vi "Picture_shrNonLin_Save_to_matlab.vi"   [LabVIEW 2011]
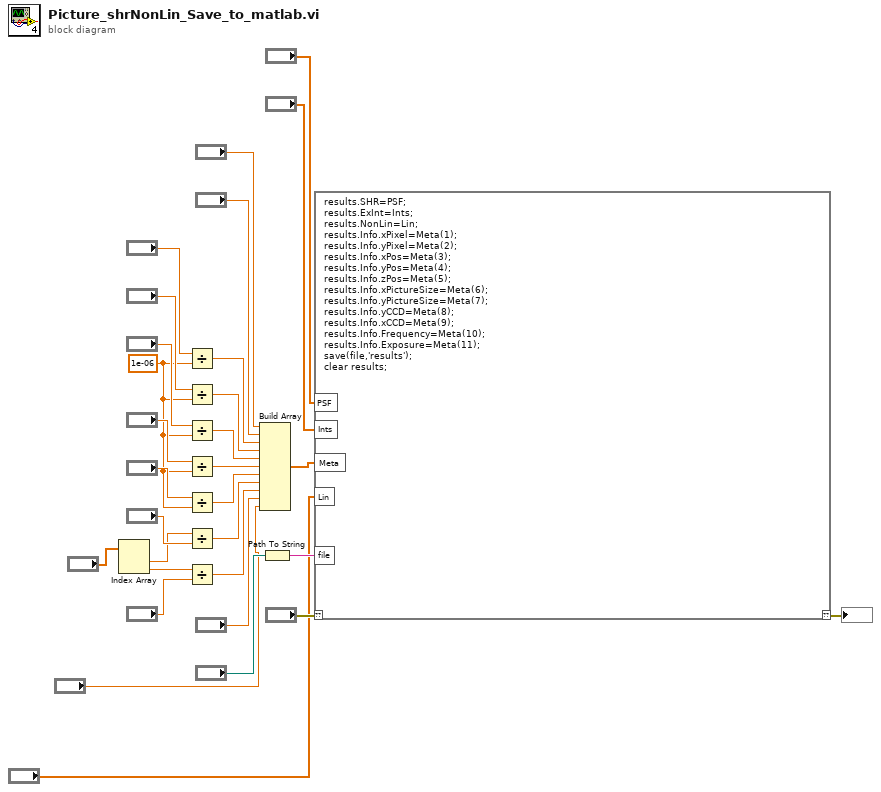
[diagram p0: block diagram]
diagram:
  w9 = 1e-06 ("y")
  n1 = Index Array(array="?") -> (element #1=w4:dbl, element #2=w5:dbl)  [unwired: 2 in]
  n2 = Divide(x="?", y=w9) -> (x/y=w22:dbl)
  n3 = Divide(x="?", y=w9) -> (x/y=w21:dbl)
  n4 = Divide(x="?", y=w9) -> (x/y=w24:dbl)
  n5 = Divide(x="?", y=w9) -> (x/y=w23:dbl)
  n6 = Divide(x="?", y=w9) -> (x/y=w25:dbl)
  n7 = Divide(x=w4, y="?") -> (x/y=w26:dbl)
  n8 = Divide(x=w5, y="?") -> (x/y=w27:dbl)
  n9 = Build Array("?", "?", w22, w21, w24, w23, w25, w26, w27, "?", "?") -> (w28:dbl[])
  n10 = Path To String(path="?") -> (string=w29:string)
  n11 = script code="results.SHR=PSF;\nresults.ExInt=Ints;\nresults.NonLin=Lin;\nresults.Info.xPixel=Meta(1);\nresults.Info.yPixel=Meta(2);\nresults.Info.xPos=Meta(3);\nresults.Info.yPos=Meta(4);\nresults.Info.zPos=Meta(5);\nresults.Info.xPictureSize=Meta(6);\nresults.Info.yPictureSize=Meta(7);\nresults.Info.yCCD=Meta(8);\nresults.Info.xCCD=Meta(9);\nresults.Info.Frequency=Meta(10);\nresults.Info.Exposure=Meta(11);\nsave(file,'results');\nclear results;"("??"="?", "PSF"="?", "Ints"="?", "Meta"=w28, "file"=w29, "Lin"="?") -> ("??"=→"?":errorcluster)
